vi "calulator for personal cal.vi"() -> ()   [LabVIEW 2020]
uses:
  <instrlib>/niRegi/niRegi.llb/niRegi Location.ctl
  <instrlib>/argus/regMaps/argus Register Maps.ctl
  <instrlib>/niRegi/niRegi.llb/niRegi Open (Regi Tag).vi
  <instrlib>/niRegi/niRegi.llb/niRegi Flush Storage Map.vi
  <vilib>/Analysis/NI_AALPro.lvlib
  <resource>/objmgr/argus/CalibrationStorageMap.rc
panel:
  in  "Overwrite to above control?":bool=TRUE
  in  "PROGRAM IN/COMMIT to cal constant":bool=TRUE
  in  "CurrentGains":u32[](array[numeric])=[4200723, 6024222]
  in  "CurrentOffset":i32[](array[numeric])=[5843724, 4041800]
  in  "VoltageGains":u32[](array[numeric])=[3896885, 3893689]
  in  "VoltageOffset":i32[](array[numeric])=[-6696216, -6515398]
  in  "Device Name 2":refnum<k21>="PXI2Slot3"
  out "stroragemap cal":errorcluster
  out "6V Offset Constant 4":i64=-6696216
  out "60V Offset Constant 3":i64=-6515398
  out "4A Offset Constant 2":i64=5843724
  out "40A Offset Constant":i64=4041800
  out "6V gain Const 4":u64=3896885
  out "60V gain Const 3":u64=3893689
  out "4A gain Const 2":u64=4200723
  out "40A gain Const":u64=6024222
  out "slope 4":dbl=0.9910291635612737
  out "intercept 4":dbl=-0.002338626575156737
  out "slope 3":dbl=0.990216259189308
  out "intercept 3":dbl=-0.022754765466275306
  out "slope 2":dbl=0.9970793882917948
  out "intercept 2":dbl=0.0013605979152736022
  out "intercept":dbl=0.009410548086866578
  out "slope":dbl=1.0213591737204284
  in  "6V":dbl[](array[numeric])=[0.103265, 5.04762]
  in  "60V range":dbl[](array[numeric])=[1.03286, 50.517]
  in  "4A range":dbl[](array[numeric])=[0.5001, 2.90713]
  in  "40A range":dbl[](array[numeric])=[0.48033, 2.83014]
  # "6V"
  # "60V"
  # "4A"
  # "40A"
  # "0.5A"
  # "3A"
  # "low"
  # "high"
  # "0.5A"
  # "3A"
  # "1V"
  # "50V"
  # "0.1V"
  # "5V"
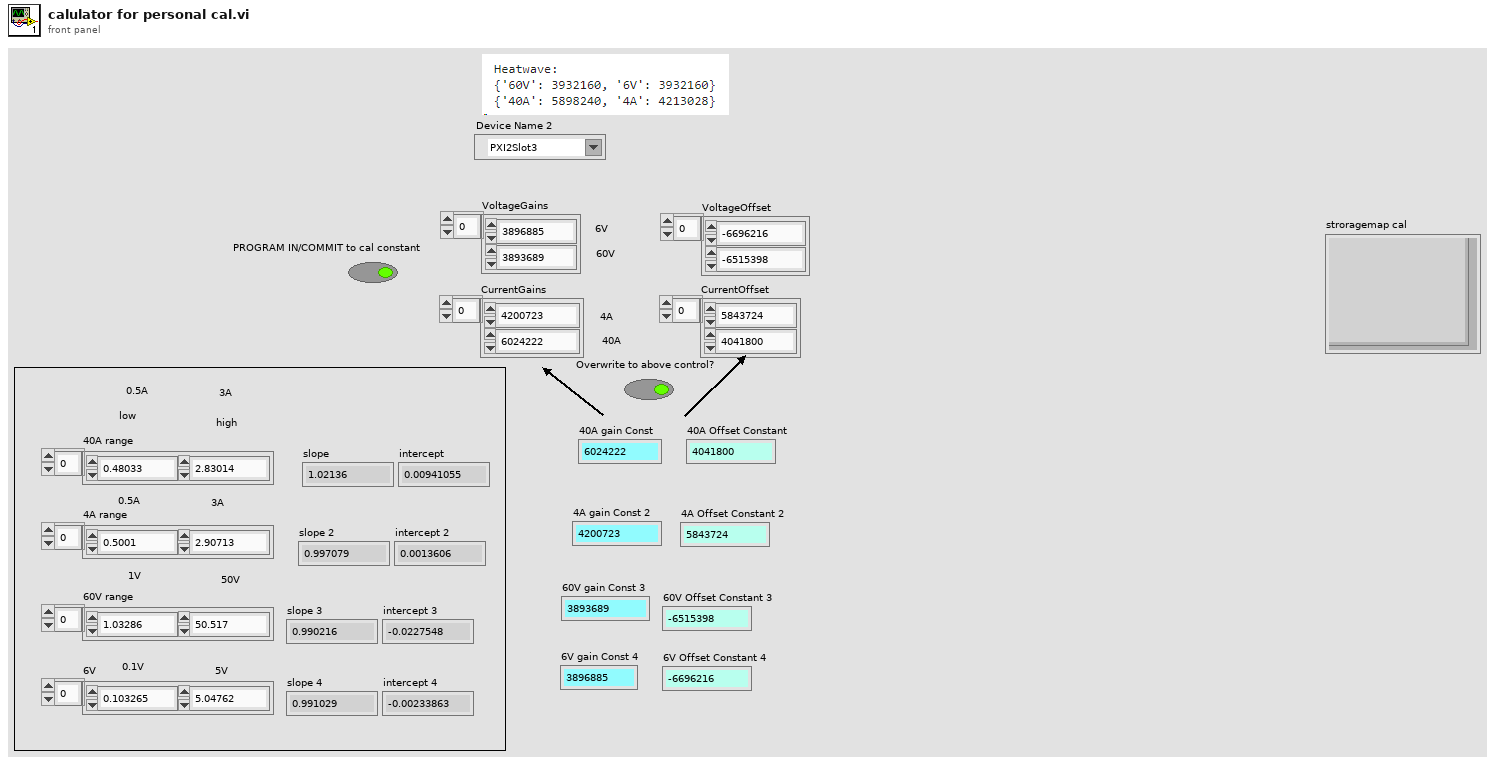
[diagram p1: front panel]
types:
  T1 = typedef "argus Register Maps.ctl" = string
  T2 = typedef "niRegi Location.ctl" = u32
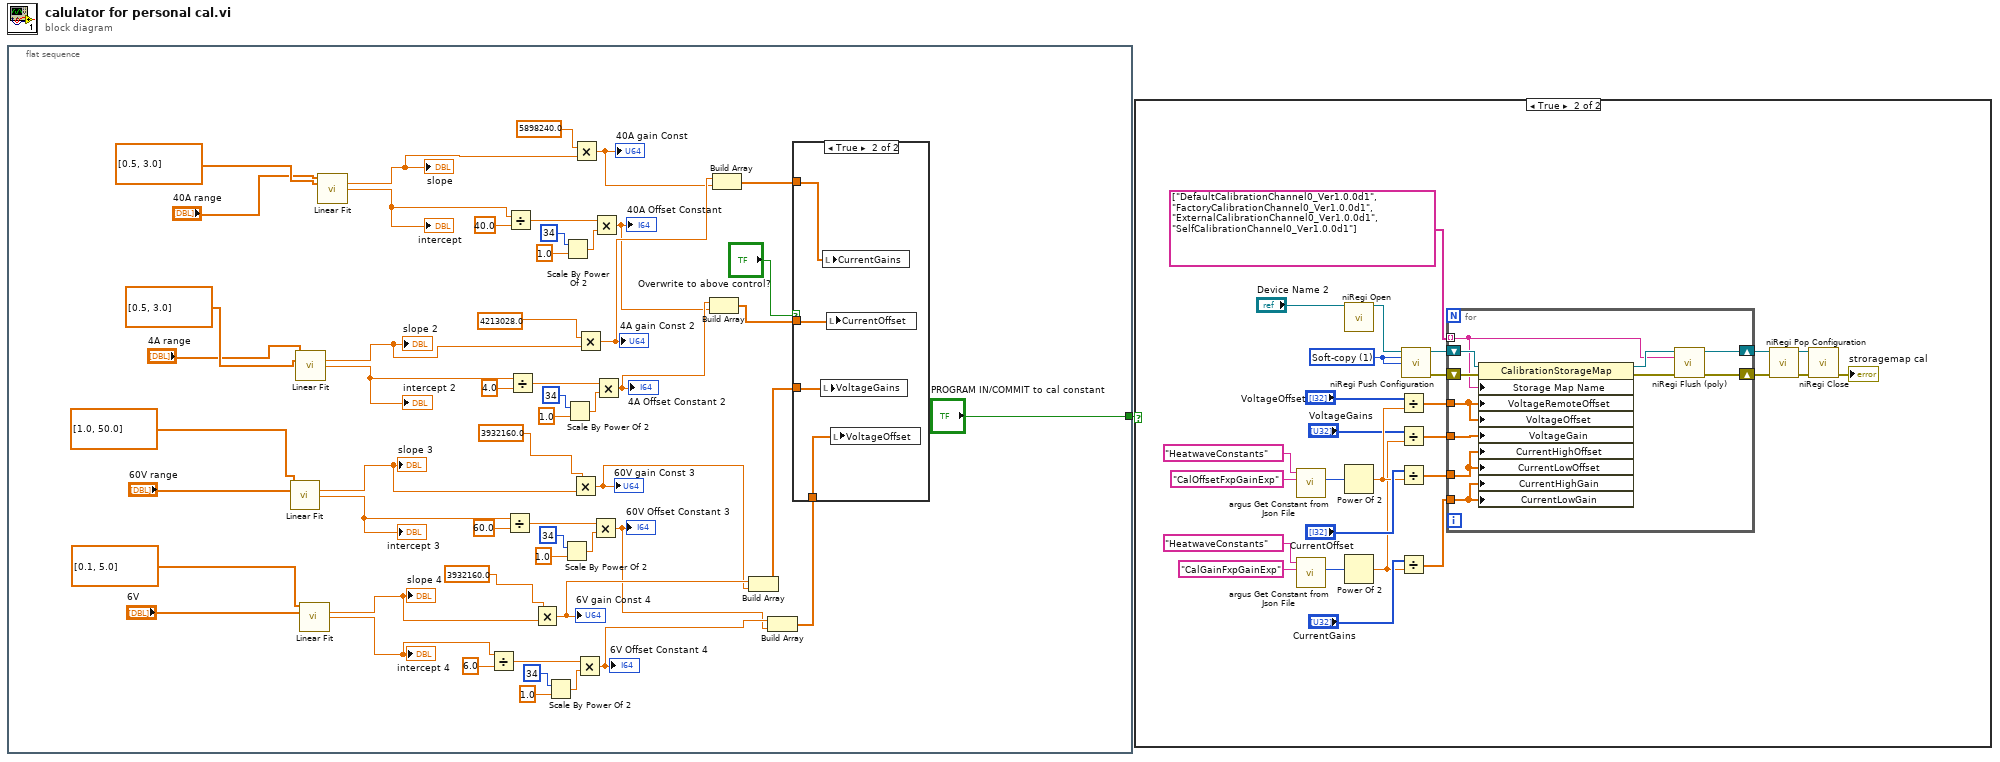
[diagram p0: block diagram]
diagram:
  n1 = flat-sequence {
    tunnel: ["PROGRAM IN/COMMIT to cal constant"] -> w1
    frame #0 {
      n2 = call <vilib>:"Linear Fit.vi"("Y"=dbl[] [1.0, 50.0], "X"="60V range") -> ("slope"=w47:dbl, "intercept"=w26:dbl)  [unwired: 9 in, 3 out]
      "slope 3" <- w47
      "intercept 3" <- w26
      n3 = call <vilib>:"Linear Fit.vi"("Y"="4A range", "X"=dbl[] [0.5, 3.0]) -> ("slope"=w46:dbl, "intercept"=w24:dbl)  [unwired: 9 in, 3 out]
      "slope 2" <- w46
      "intercept 2" <- w24
      n4 = call <vilib>:"Linear Fit.vi"("Y"=dbl[] [0.1, 5.0], "X"="6V") -> ("slope"=w49:dbl, "intercept"=w28:dbl)  [unwired: 9 in, 3 out]
      "slope 4" <- w49
      "intercept 4" <- w28
      n5 = call <vilib>:"Linear Fit.vi"("Y"="40A range", "X"=dbl[] [0.5, 3.0]) -> ("slope"=w50:dbl, "intercept"=w22:dbl)  [unwired: 9 in, 3 out]
      "slope" <- w50
      "intercept" <- w22
      n6 = Divide(x=w28, y=6.0) -> (x/y=w29:dbl)
      n7 = Divide(x=w26, y=60.0) -> (x/y=w36:dbl)
      n8 = Divide(x=w22, y=40.0) -> (x/y=w44:dbl)
      n9 = Divide(x=w24, y=4.0) -> (x/y=w37:dbl)
      n10 = Multiply(x=3932160.0, y=w49) -> (x*y=w20:dbl)
      "6V gain Const 4" <- w20
      n11 = Scale By Power Of 2(n=i16 34, x=1.0) -> (x*2^n=w30:dbl)
      n12 = Scale By Power Of 2(n=i16 34, x=1.0) -> (x*2^n=w35:dbl)
      n13 = Scale By Power Of 2(n=i16 34, x=1.0) -> (x*2^n=w43:dbl)
      n14 = Scale By Power Of 2(n=i16 34, x=1.0) -> (x*2^n=w38:dbl)
      n15 = Multiply(x=3932160.0, y=w47) -> (x*y=w16:dbl)
      "60V gain Const 3" <- w16
      n16 = Multiply(x=5898240.0, y=w50) -> (x*y=w11:dbl)
      "40A gain Const" <- w11
      n17 = Multiply(x=w29, y=w30) -> (x*y=w15:dbl)
      "6V Offset Constant 4" <- w15
      n18 = Multiply(x=4213028.0, y=w46) -> (x*y=w12:dbl)
      "4A gain Const 2" <- w12
      n19 = Multiply(x=w36, y=w35) -> (x*y=w14:dbl)
      "60V Offset Constant 3" <- w14
      n20 = Multiply(x=w44, y=w43) -> (x*y=w8:dbl)
      "40A Offset Constant" <- w8
      n21 = Multiply(x=w37, y=w38) -> (x*y=w9:dbl)
      "4A Offset Constant 2" <- w9
      n22 = Build Array(w9, w8) -> (w7:dbl[])
      n23 = Build Array(w12, w11) -> (w10:dbl[])
      n24 = Build Array(w20, w16) -> (w17:dbl[])
      n25 = Build Array(w15, w14) -> (w13:dbl[])
      n26 = case shown="True" "Overwrite to above control?" {
        tunnel: w17 -> [_ w59]
        tunnel: w13 -> [_ w58]
        tunnel: w10 -> [_ w57]
        tunnel: w7 -> [_ w56]
        frame False {
        }
        frame True {
          n27 = local write "VoltageGains"(w59) -> ()
          n28 = local write "CurrentGains"(w57) -> ()
          n29 = local write "CurrentOffset"(w56) -> ()
          n30 = local write "VoltageOffset"(w58) -> ()
        }
      }
    }
  }
  n31 = case shown="True" w1 {
    frame False {
    }
    frame True {
      w60 = T2 1 items=["Keep Current Cfg"=4294967295, "Hardware"=0, "Soft-copy"=1] ("Write Destination")
      n32 = call <instrlib>:"argus Get Constant from Json File.vi"("Constant Name"="CalOffsetFxpGainExp", "Register Map"=T1 "HeatwaveConstants") -> ("Constant Value"=w80:i32)  [unwired: 9 in]
      n33 = call <instrlib>:"argus Get Constant from Json File.vi"("Constant Name"="CalGainFxpGainExp", "Register Map"=T1 "HeatwaveConstants") -> ("Constant Value"=w75:i32)  [unwired: 9 in]
      n34 = call-poly <instrlib>:"niRegi Open.vi"("Device Name"="Device Name 2") -> ("Regi Session"=w66:refnum<k21>)  [unwired: 13 in, 1 out]
      n35 = Power Of 2(x=w80) -> (2^x=w83:dbl)
      n36 = Power Of 2(x=w75) -> (2^x=w78:dbl)
      n37 = Divide(x="VoltageOffset", y=w83) -> (x/y=w82:dbl[])
      n38 = Divide(x="VoltageGains", y=w78) -> (x/y=w77:dbl[])
      n39 = Divide(x="CurrentOffset", y=w83) -> (x/y=w85:dbl[])
      n40 = Divide(x="CurrentGains", y=w78) -> (x/y=w86:dbl[])
      n41 = call <instrlib>:"niRegi Push Configuration.vi"("Regi Session"=w66, "Read Source"=w60, "Write Destination"=w60) -> ("Regi Session Out"=w67:refnum<k21>, "error out"=w68:errorcluster)  [unwired: 11 in]
      n42 = for {
        shift-right: [w97] -> w71
        shift-left: w68 -> [w95]
        shift-right: [w96] -> w72
        shift-left: w67 -> [w92]
        tunnel: string[] ["DefaultCalibrationChannel0_Ver1.0.0d1", "FactoryCalibrationChannel0_Ver1.0.0d1", "ExternalCalibrationChannel0_Ver1.0.0d1", "SelfCalibrationChannel0_Ver1.0.0d1"] ("Storage Map Name") -> [w87] mode=indexing
        tunnel: w77 -> [w91]
        tunnel: w86 -> [w90]
        tunnel: w82 -> [w89]
        tunnel: w85 -> [w88]
        n43 = property class="CalibrationStorageMap"(reference=w92, error in=w95, "Storage Map Name"=w87, "VoltageRemoteOffset"=w89, "VoltageOffset"=w89, "VoltageGain"=w91, "CurrentHighOffset"=w88, "CurrentLowOffset"=w88, "CurrentHighGain"=w90, "CurrentLowGain"=w90) -> (reference out=w93:refnum<k21>, error out=w94:errorcluster)
        n44 = call-poly <instrlib>:"niRegi Flush (poly).vi"("Regi Session"=w93, "Storage Map (*)"=w87, "error in"=w94) -> ("Regi Session Out"=w96:refnum<k21>, "error out"=w97:errorcluster)  [unwired: 11 in]
      }
      n45 = call <instrlib>:"niRegi Pop Configuration.vi"("Regi Session"=w72, "error in"=w71) -> ("Regi Session Out"=w69:refnum<k21>, "error out"=w70:errorcluster)  [unwired: 9 in, 3 out]
      n46 = call <instrlib>:"niRegi Close.vi"("Regi Session"=w69, "error in"=w70) -> ("error out"=→"stroragemap cal":errorcluster)  [unwired: 13 in]
    }
  }
